vi "Fault.vi"(8 "error in (no error)":errorcluster, 11 "VISA resource name":refnum<visa-resource-name>) -> (0 "error out":errorcluster, 1 "Fault Value (string)":string, 2 "Fault Value (integer)":i32, 3 "VISA resource name out":refnum<visa-resource-name>)   [LabVIEW 2021, in "Sorensen M9A Series.lvlib"]
doc: "This VI returns the integer value of the fault register for the fault condition status."
uses:
  Sorensen M9A Series.lvlib
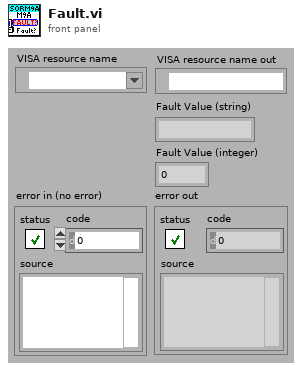
[diagram p1: front panel]
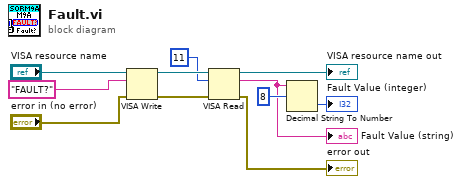
[diagram p0: block diagram]
diagram:
  n1 = VISA Write(VISA resource name="VISA resource name", write buffer="FAULT?" ("data"), error in (no error)="error in (no error)") -> (VISA resource name out=w6:refnum<visa-resource-name>, error out=w5:errorcluster)  [unwired: 1 out]
  n2 = VISA Read(VISA resource name=w6, byte count=11, error in (no error)=w5) -> (VISA resource name out=→"VISA resource name out":refnum<visa-resource-name>, read buffer=w3:string, error out=→"error out":errorcluster)  [unwired: 1 out]
  "Fault Value (string)" <- w3
  n3 = Decimal String To Number(string=w3, offset=8) -> (number=→"Fault Value (integer)":i32)  [unwired: 1 in, 1 out]
